vi "Resolve Local File.vi"(8 "error in (no error)":errorcluster, 10 "Request Path":string, 11 "StandardFileServe in":refnum<class "StandardFileServe.lvclass">) -> (0 "error out":errorcluster, 2 "Path":path, 3 "StandardFileServe out":refnum<class "StandardFileServe.lvclass">)   [LabVIEW 2020, in "HTTP Server.lvlib" / "StandardFileServe.lvclass"]
uses:
  StandardFileServe.lvclass
  StandardFileServe.lvclass/StandardFileServe.ctl
  lv-uri/URI/URI.lvlib
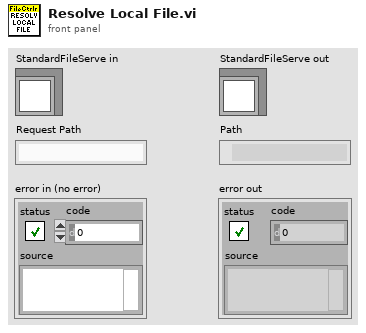
[diagram p1: front panel]
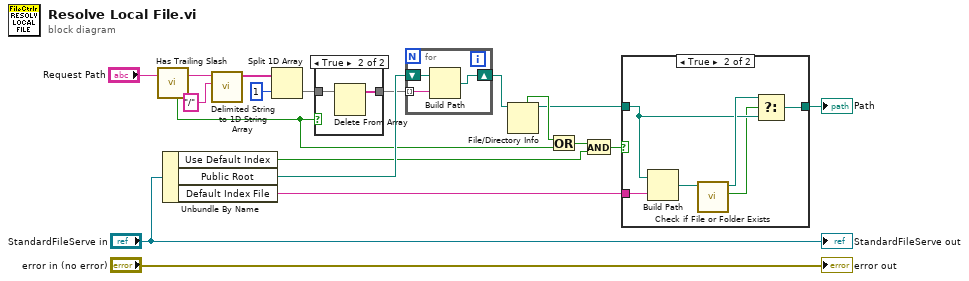
[diagram p0: block diagram]
diagram:
  n1 = call "Has Trailing Slash.vi"("Path String in"="Request Path") -> ("Has Trailing Slash"=w6:bool, "Path String"=w16:string)  [unwired: 5 in]
  n2 = Unbundle By Name("StandardFileServe in") -> ("Use Default Index"=w4:bool, "Public Root"=w10:path, "Default Index File"=w11:string)
  n3 = call <vilib>:"Delimited String to 1D String Array.vi"("delimiter"="/", "delimited string"=w16) -> ("string array"=w14:string[])  [unwired: 9 in]
  n4 = Split 1D Array(array=w14, index=1) -> (second subarray=w12:string[])  [unwired: 1 out]
  n5 = case shown="True" w6 {
    tunnel: w12 -> [w20 w22]
    tunnel: [w20 w21] -> w9
    frame False {
    }
    frame True {
      n6 = Delete From Array(array=w22) -> (array with subset deleted=w21:string[])  [unwired: 2 in, 1 out]
    }
  }
  n7 = for {
    shift-right: [w24] -> w8
    shift-left: w10 -> [w25]
    tunnel: w9 -> [w23] mode=indexing
    n8 = Build Path(base path=w25, name or relative path=w23) -> (appended path=w24:path)
  }
  n9 = File/Directory Info(path=w8) -> (path out=w2:path, directory=w7:bool)  [unwired: 1 in, 5 out]
  n10 = Or(x=w7, y=w6) -> (x .or. y?=w5:bool)
  n11 = And(x=w5, y=w4) -> (x .and. y?=w3:bool)
  n12 = case shown="True" w3 {
    tunnel: w11 -> [_ w32]
    tunnel: w2 -> [w26 w29]
    tunnel: [w26 w28] -> w18
    frame False {
    }
    frame True {
      n13 = Build Path(base path=w29, name or relative path=w32) -> (appended path=w31:path)
      n14 = call <vilib>:"Check if File or Folder Exists.vi"("path"=w31) -> ("file or folder exists?"=w27:bool, "dup path"=w30:path)  [unwired: 8 in, 1 out]
      n15 = Select(t=w30, s=w27, f=w29) -> (s? t:f=w28:path)
    }
  }
  "Path" <- w18
  "error out" <- "error in (no error)"
  "StandardFileServe out" <- "StandardFileServe in"
